vi "Digitizer_initialization.vi"(0 "Device":i32, 1 "Triger Source":T5(ring)=enum."External", 4 "RecordLength":u32=4096, 5 "9350_Range 2":u32(ring)=3 items=["40mV", "100mV", "200mV", "400mV", "1 V", "2 V", "4 V"], 7 "samplerate":enum16{"500M", "250M", "125M"}(ring), 9 "9350_Range":u32(ring)=3 items=["40mV", "100mV", "200mV", "400mV", "1 V", "2 V", "4 V"], 11 "Channel":T3, 12 "Trig. Delay (us)":sgl=7.1, 13 "Level":u32=151, 14 "Slope":enum32{"Positive", "Negative"}(ring), 15 "Rec/Buf":u32=256) -> (2 "PLL Locked":bool, 3 "DeviceOut":i32, 10 "Error":bool)   [LabVIEW 2015]
uses:
  AlazarTech/ATS-VI/5.8.3/ATS_ctl/Coupling.ctl
  AlazarTech/ATS-VI/5.8.3/ATS_ctl/ExtTrigRange.ctl
  AlazarTech/ATS-VI/5.8.3/ATS_ctl/Impedance.ctl
  AlazarTech/ATS-VI/5.8.3/ATS_ctl/ATS_DMA_Channel.ctl
  AlazarTech/ATS-VI/5.8.3/ATS_ctl/ClockSource.ctl
  AlazarTech/ATS-VI/5.8.3/ATS_ctl/ClockRate.ctl
  AlazarTech/ATS-VI/5.8.3/ATS_ctl/Device_Ctrl.ctl
  AlazarTech/ATS-VI/5.8.3/ATS_ctl/ATS_Check_Ctrl.ctl
  AlazarTech/ATS-VI/5.8.3/ATS_ctl/ClockEdge.ctl
  AlazarTech/ATS-VI/5.8.3/ATS_ctl/TriggerOperation.ctl
  AlazarTech/ATS-VI/5.8.3/ATS_ctl/ATS_Async_Ctrl.ctl
  AlazarTech/ATS-VI/5.8.3/ATS_ctl/ATS_ReadSamples.ctl
  AlazarTech/ATS-VI/5.8.3/ATS_ctl/ATS_Async_Mode.ctl
  AlazarTech/ATS-VI/5.8.3/ATS_ctl/ATS_Async_Setting.ctl
  AlazarTech/ATS-VI/5.8.3/ATS_ctl/Bandwidth.ctl
  AlazarTech/ATS-VI/5.8.3/ATS_ctl/Clock.ctl
  ATSApi.dll
panel:
  in  "ClckRate":T1=19 items=["1 kS/s", "2 kS/s", "5 kS/s", "10 kS/s", "20 kS/s", "50 kS/s", "100 kS/s", "200 kS/s", "500 kS/s", "1 MS/s", "2 MS/s", "5 MS/s", "10 MS/s", "20 MS/s", "25 MS/s", "50 MS/s", "100 MS/s", "125 MS/s", "200 MS/s", "500 MS/s", "1 GS/s"]
  in  "BufCount":i32=16
  in  "ClckSource":T2
  in  "Impedance 2":T4=enum."50 ohms"
  in  "Impedance":T4=enum."50 ohms"
  in  "WaitTimeOut (ms)":u32=1000
  in  "Ext Trig":cluster{"Coupling":T6, "Range":T7}={"Coupling"=enum."DC", "Range"=enum."5 V"}
  out "StartCapture Status":string
  out "SetupDMA Status":string
  out "cFlags_Out":u32 format="%x"
  out "Board":string
  # "ATS9350 Simple AsynchronousDMA Initialization"
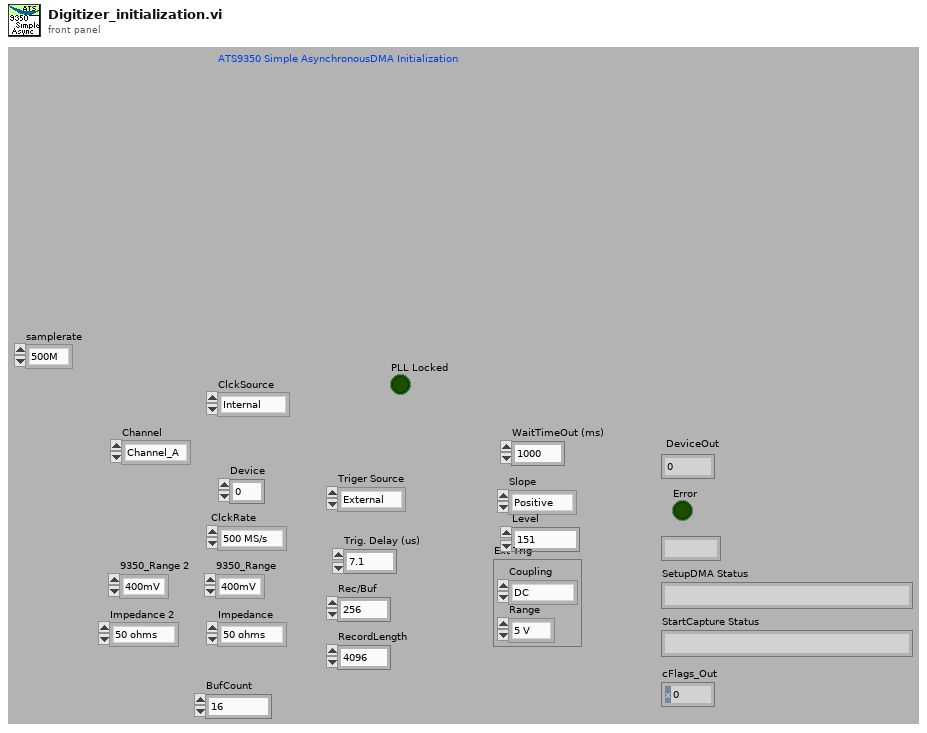
[diagram p1: front panel]
types:
  T1 = typedef "ClockRate.ctl" = u32
  T2 = typedef "ClockSource.ctl" = enum16{"Internal", "External", "Medium Ext.", "Slow Ext.", "Ext. AC", "Ext. DC", "Ext. (PLL)"}
  T3 = typedef "ATS_DMA_Channel.ctl" = enum16{"Channel_A", "Channel_B", "A & B"}
  T4 = typedef "Impedance.ctl" = enum16{"1M ohms", "50 ohms"}
  T5 = enum32{"Chan_A", "Chan_B", "External", "Disable"}
  T6 = typedef "Coupling.ctl" = enum16{"AC", "DC"}
  T7 = typedef "ExtTrigRange.ctl" = enum16{"1 V", "5 V"}
  T8 = typedef "ATS_Async_Ctrl.ctl" = enum16{"SetupDMA", "StartCapture", "Get", "Get_Stream", "Abort", "Stop"}
  T9 = typedef "ATS_Async_Setting.ctl" = cluster{"UseHeader":u32, "Rec/Buffer":u32, "Total_Rec":u32, "DataBuffer":bool, "GetProcessedData":bool}
  T10 = typedef "ATS_Async_Mode.ctl" = enum16{"Continuous", "Triggered", "No-Pre-Trigger", "Traditional"}
  T11 = typedef "ATS_ReadSamples.ctl" = cluster{"Offset":i32, "Length":u32}
  T12 = typedef "ATS_Check_Ctrl.ctl" = enum16{"None", "NO_ATS9462", "ATS9462_Traditional", "Verify Board", "OnBoard Memory", "Board & Memory"}
  T13 = typedef "Device_Ctrl.ctl" = enum16{"Status", "About", "Arm", "ForceTrig", "Abort", "Initialize", "Init (NoPreset)", "Info", "Close", "Calibrate", "SetManually", "LED_ON", "LED_OFF"}
  T14 = typedef "Clock.ctl" = cluster{"ClckSource":T2, "ClckRate":T1, "ClckEdge":T15, "Decimation":u32}
  T15 = typedef "ClockEdge.ctl" = u16
  T16 = typedef "Bandwidth.ctl" = enum16{"Full Bandwidth", "Reduce Bandwidth"}
  T17 = cluster{"Source":enum32{"Chan_A", "Chan_B", "External", "Disable"}, "Slope":enum32{"Positive", "Negative"}, "Level":u32}
  T18 = typedef "TriggerOperation.ctl" = enum16{"Only X", "Only Y", "X or Y", "X and Y", "X xor Y", "X and not Y", "not X and Y"}
  T19 = cluster{"Triger Source":enum32{"Chan_A", "Chan_B", "External", "Disable"}, "Slope":enum32{"Positive", "Negative"}, "Level":u32}
  T20 = cluster{"Engine Relationship":T18, "Timeout (s)":dbl, dbl, cluster{"Triger Source":enum32{"Chan_A", "Chan_B", "External", "Disable"}, "Slope":enum32{"Positive", "Negative"}, "Level":u32}, "EngineY":cluster{"Source":enum32{"Chan_A", "Chan_B", "External", "Disable"}, "Slope":enum32{"Positive", "Negative"}, "Level":u32}, "Ext Trig":cluster{"Coupling":T6, "Range":T7}}
  T21 = cluster{"ClckSource":T2, "ClckRate":T1, "ClckEdge":T15, "Decimation":u32}
  T22 = cluster{"Coupling":T6, "9350_Range":u32, "Impedance":T4, "Bandwidth":T16}
  T23 = cluster{"Coupling":T6, "9350_Range 2":u32, "Impedance 2":T4, "Bandwidth":T16}
  T24 = typedef "Device_Info.ctl" = cluster{"Handle":u32, "Board":string, "CPLD":string, "MemorySize":u32, "SampleSize":u8, "ID":i32, "High_Memory":bool}
  T25 = cluster{"Count":cluster{"Count":u32, "Offset":i32, "Length":u32}, cluster{"ClckSource":T2, "ClckRate":T1, "ClckEdge":T15, "Decimation":u32}, cluster{"Coupling":T6, "9350_Range":u32, "Impedance":T4, "Bandwidth":T16}, cluster{"Coupling":T6, "9350_Range 2":u32, "Impedance 2":T4, "Bandwidth":T16}, cluster{"Engine Relationship":T18, "Timeout (s)":dbl, dbl, cluster{"Triger Source":enum32{"Chan_A", "Chan_B", "External", "Disable"}, "Slope":enum32{"Positive", "Negative"}, "Level":u32}, "EngineY":cluster{"Source":enum32{"Chan_A", "Chan_B", "External", "Disable"}, "Slope":enum32{"Positive", "Negative"}, "Level":u32}, "Ext Trig":cluster{"Coupling":T6, "Range":T7}}}
  T26 = typedef "ATS_Async_Status.ctl" = cluster{"Start DMA":bool, "StartCapture":bool, "Valid":bool, "Completed":bool, "InProgress":bool, "Timeout":bool, "Overflow":bool, "Error":bool}
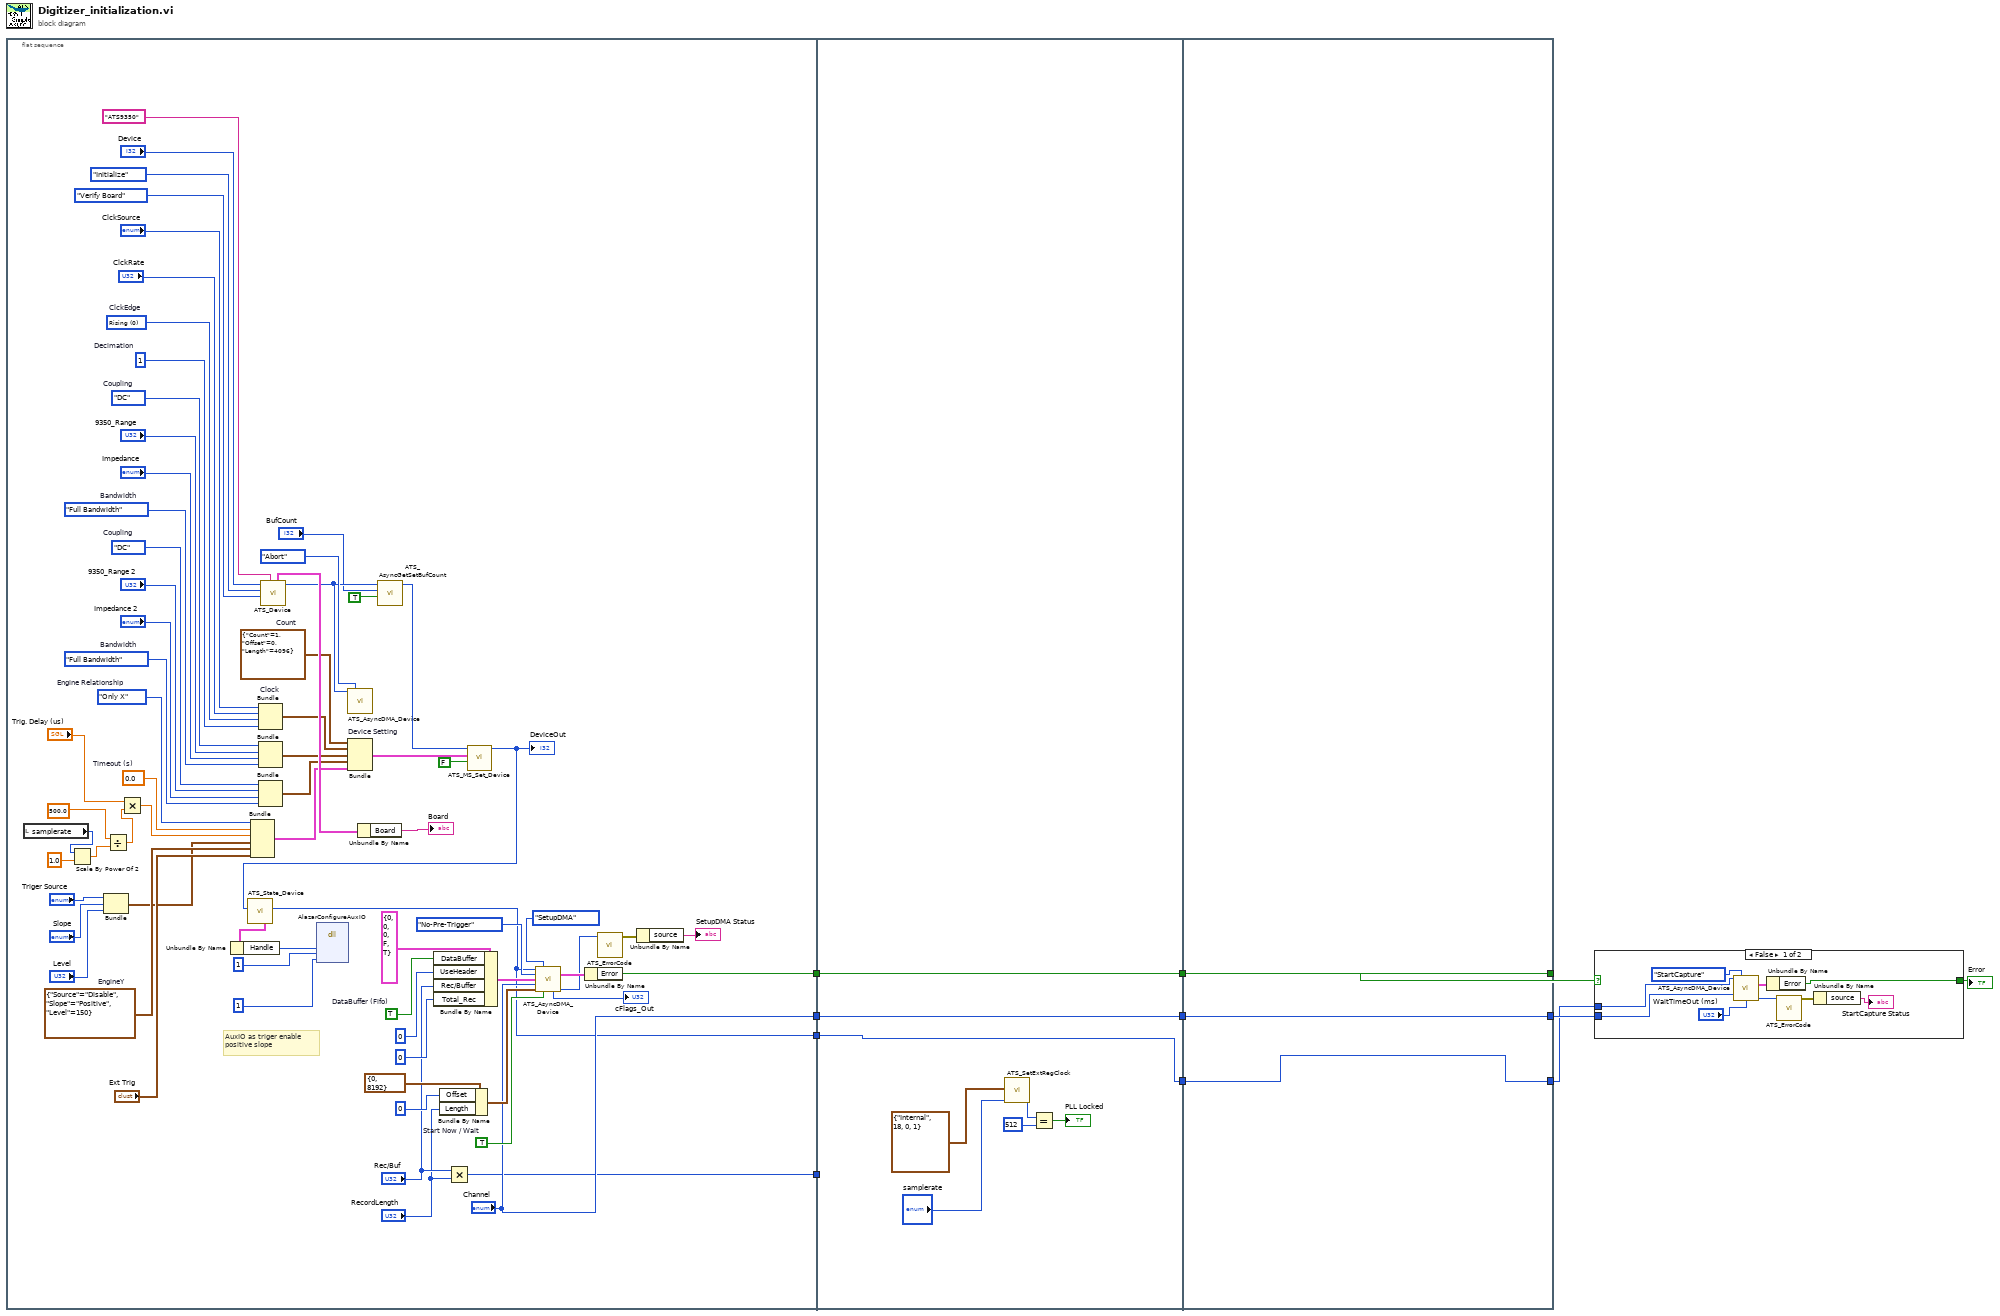
[diagram p0: block diagram]
diagram:
  n1 = flat-sequence {
    tunnel: [w48] -> w7
    tunnel: ["Channel"] -> w6
    tunnel: [w24] -> w5
    tunnel: [w17] -> w4
    tunnel: w7 -> [w91]
    tunnel: w6 -> [w90]
    tunnel: w5 -> [w84]
    tunnel: w4 -> [_]
    tunnel: [w91] -> w3
    tunnel: [w90] -> w2
    tunnel: [w84] -> w1
    tunnel: [w92] -> w8
    tunnel: [w93] -> w9
    tunnel: [w94] -> w10
    tunnel: w3 -> [w94]
    tunnel: w2 -> [w93]
    tunnel: w1 -> [w92]
    frame #0 {
      w39 = Bandwidth."Full Bandwidth"  # Bandwidth
      w40 = Coupling."DC"  # Coupling
      w50 = TRUE  # DataBuffer (Fifo)
      w63 = TRUE  # Start Now / Wait
      w68 = T17 {"Source"=enum."Disable", "Slope"=enum."Positive", "Level"=150}  # EngineY
      w69 = cluster{"Count":u32, "Offset":i32, "Length":u32} {"Count"=1, "Offset"=0, "Length"=4096}  # Count
      w70 = Bandwidth."Full Bandwidth"  # Bandwidth
      w71 = u32 1  # Decimation
      w76 = TriggerOperation."Only X"  # Engine Relationship
      w77 = 0.0  # Timeout (s)
      w74 = Coupling."DC"  # Coupling
      w75 = T15 0 items=["Rising", "Falling"]  # ClckEdge
      # "AuxIO as triger enable\npositive slope"
      n2 = local read "samplerate"() -> (w15:enum16{"500M", "250M", "125M"})
      n3 = Scale By Power Of 2(n=w15, x=1.0) -> (x*2^n=w13:dbl)
      n4 = Bundle("Triger Source"="Triger Source", "Slope"="Slope", "Level"="Level") -> (w42:T19)  [unwired: 1 out]
      n5 = Divide(x=sgl 500.0 ("y"), y=w13) -> (x/y=w12:dbl)
      n6 = Multiply(x="Trig. Delay (us)", y=w12) -> (x*y=w46:dbl)
      n7 = Bundle("Engine Relationship"=w76, "Timeout (s)"=w77, w46, w42, "EngineY"=w68, "Ext Trig"="Ext Trig") -> (w72:T20)  [unwired: 1 out]
      n8 = Bundle "Clock"("ClckSource"="ClckSource", "ClckRate"="ClckRate", "ClckEdge"=w75, "Decimation"=w71) -> (w27:T21)  [unwired: 1 out]
      n9 = Bundle("Coupling"=w74, "9350_Range"="9350_Range", "Impedance"="Impedance", "Bandwidth"=w70) -> (w73:T22)  [unwired: 1 out]
      n10 = Bundle("Coupling"=w40, "9350_Range 2"="9350_Range 2", "Impedance 2"="Impedance 2", "Bandwidth"=w39) -> (w37:T23)  [unwired: 1 out]
      n11 = call "ATS_Device.vi"("BoardToVerify"="ATS9350", "ATS_Check"=ATS_Check_Ctrl."Verify Board", "DevCtrl"=Device_Ctrl."Initialize", "DeviceIn"="Device") -> ("DeviceOut"=w31:i32, "DevInfo"=w78:T24)  [unwired: 1 in, 5 out]
      n12 = call "ATS_AsyncDMA_Device.vi"("DeviceIn"=w31, "ATS_Async_Ctrl"=ATS_Async_Ctrl."Abort") -> ()  [unwired: 6 in, 8 out]
      n13 = Bundle "Device Setting"("Count"=w69, w27, w73, w37, w72) -> (w66:T25)  [unwired: 1 out]
      n14 = Unbundle By Name(w78) -> ("Board"=→"Board":string)
      n15 = call "ATS_AsyncGetSetBufCount.vi"("Get / Set&Get"=TRUE, "BuffCount"="BufCount", "DeviceIn"=w31) -> ("DeviceOut"=w28:i32)  [unwired: 8 out]
      n16 = Bundle By Name(cluster=T9 {"UseHeader"=0, "Rec/Buffer"=0, "Total_Rec"=0, "DataBuffer"=FALSE, "GetProcessedData"=TRUE} ("Async_Setting"), "DataBuffer"=w50, "UseHeader"=u32 0, "Rec/Buffer"="Rec/Buf", "Total_Rec"=u32 0 ("Records")) -> (w62:T9)
      n17 = Bundle By Name(cluster=T11 {"Offset"=0, "Length"=8192} ("Trad_ReadSamples"), "Offset"=0, "Length"="RecordLength") -> (w58:T11)
      n18 = Multiply(x="Rec/Buf", y="RecordLength") -> (x*y=w17:u32)
      n19 = call "ATS_MS_Set_Device.vi"("Set_Manually (F)"=FALSE, "Setup_In"=w66, "DeviceIn"=w28) -> ("DeviceOut"=w25:i32)  [unwired: 1 in, 7 out]
      "DeviceOut" <- w25
      n20 = call "ATS_State_Device.vi"("DeviceIn"=w25) -> ("DeviceOut"=w24:i32, "DevInfo_Out"=w23:T24)  [unwired: 5 in, 4 out]
      n21 = Unbundle By Name(w23) -> ("Handle"=w22:u32)
      n22 = dll-call lib="ATSApi.dll" fn="AlazarConfigureAuxIO"("handle"=w22, "mode"=1, "para"=1) -> ()  [unwired: 7 in, 2 out]
      n23 = call "ATS_AsyncDMA_Device.vi"("DeviceIn"=w24, "ATS_Async_Ctrl"=ATS_Async_Ctrl."SetupDMA" ("ATS_DMA_Ctrl"), "Async_Mode"=ATS_Async_Mode."No-Pre-Trigger", "Async_Setting"=w62, "Channel"="Channel", "ReadSamples"=w58, "Start Now / Wait"=w63) -> ("Async_Status"=w54:T26, "cFlags_Out"=→"cFlags_Out":u32, "Return Code"=w52:u32)  [unwired: 1 in, 5 out]
      n24 = Unbundle By Name(w54) -> ("Error"=w48:bool)
      n25 = call "ATS_ErrorCode.vi"("ErrorCode"=w52) -> ("error out"=w53:errorcluster)  [unwired: 1 in, 5 out]
      n26 = Unbundle By Name(w53) -> ("source"=→"SetupDMA Status":string)
    }
    frame #1 {
      n27 = call "ATS_SetExtRegClock.vi"("rate"="samplerate", "Clock"=T14 {"ClckSource"=enum."Internal", "ClckRate"=18, "ClckEdge"=0, "Decimation"=1}) -> ("Return Code"=w88:u32)  [unwired: 1 in, 8 out]
      n28 = Equal?(x=w88, y=u32 512) -> (x = y?=→"PLL Locked":bool)
    }
    frame #2 {
    }
  }
  n29 = case shown="False" w10 {
    selector: w10 -> [_ w104]
    tunnel: [w98 w104] -> w11
    tunnel: w8 -> [w97 _]
    tunnel: w9 -> [w95 _]
    frame False {
      n30 = call "ATS_AsyncDMA_Device.vi"("DeviceIn"=w97, "ATS_Async_Ctrl"=ATS_Async_Ctrl."StartCapture", "Channel"=w95, "WaitTimeOut (ms)"="WaitTimeOut (ms)") -> ("Async_Status"=w100:T26, "Return Code"=w102:u32)  [unwired: 4 in, 6 out]
      n31 = Unbundle By Name(w100) -> ("Error"=w98:bool)
      n32 = call "ATS_ErrorCode.vi"("ErrorCode"=w102) -> ("error out"=w101:errorcluster)  [unwired: 1 in, 5 out]
      n33 = Unbundle By Name(w101) -> ("source"=→"StartCapture Status":string)
    }
    frame True {
    }
  }
  "Error" <- w11
